vi "TurnOn.vi"(7 "Voltage Set (V)":dbl, 8 "error in (no error)":errorcluster, 9 "OCP Level (A)":dbl, 10 "OVP Level (V)":dbl, 11 "PSU_N87 in":refnum<class "PSU_N87.lvclass">) -> (0 "error out":errorcluster, 3 "PSU_N87 out":refnum<class "PSU_N87.lvclass">)   [LabVIEW 2014, in "PSU_N87.lvclass"]
uses:
  PSU_N87.lvclass
  PSU_N87.lvclass/PSU_N87.ctl
  PSU.lvclass
  <instrlib>/Agilent N87XX Series/Agilent N87XX Series.lvlib
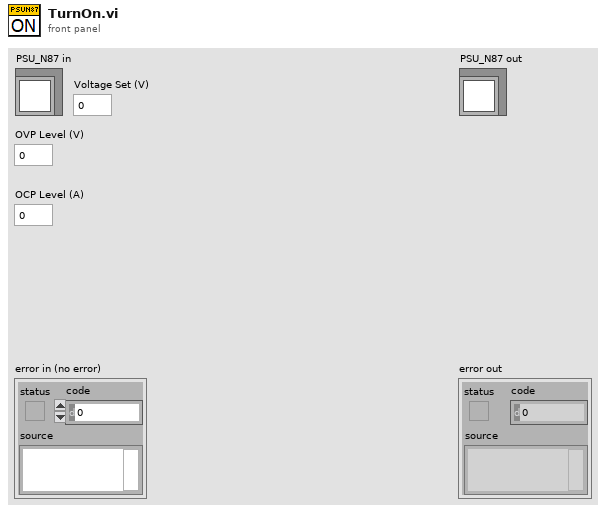
[diagram p1: front panel]
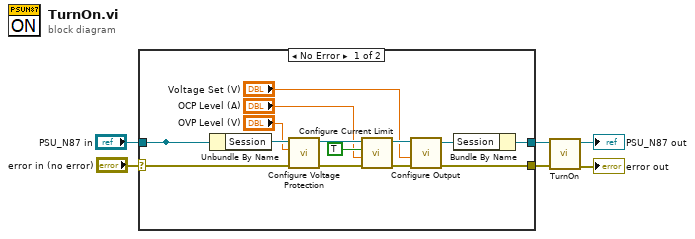
[diagram p0: block diagram]
diagram:
  n1 = case shown="No Error" "error in (no error)" {
    selector: "error in (no error)" -> [w15 w22]
    tunnel: [w14 w22] -> w3
    tunnel: "PSU_N87 in" -> [w12 w21]
    tunnel: [w7 w21] -> w4
    frame No Error {
      n2 = Unbundle By Name(w12) -> ("Session"=w13:refnum<visa-resource-name>)
      n3 = call <instrlib>:"Configure Voltage Protection.vi"("error in (no error)"=w15, "Over-Voltage Protection (5.0 V)"="OVP Level (V)", "VISA resource name"=w13) -> ("error out"=w16:errorcluster, "VISA resource name out"=w17:refnum<visa-resource-name>)  [unwired: 7 in]
      n4 = call <instrlib>:"Configure Current Limit.vi"("error in (no error)"=w16, "Current Limit (0.0 A)"="OCP Level (A)", "Enable Current Protection (F: Disable)"=TRUE, "VISA resource name"=w17) -> ("error out"=w18:errorcluster, "VISA resource name out"=w19:refnum<visa-resource-name>)  [unwired: 6 in]
      n5 = call <instrlib>:"Configure Output.vi"("error in (no error)"=w18, "Voltage Level (0.0 V)"="Voltage Set (V)", "VISA resource name"=w19) -> ("error out"=w14:errorcluster, "VISA resource name out"=w11:refnum<visa-resource-name>)  [unwired: 7 in]
      n6 = Bundle By Name(cluster=w12, "Session"=w11) -> (w7:refnum<class "PSU_N87.lvclass">)
    }
    frame Error {
    }
  }
  n7 = call-parent "TurnOn.vi"("error in (no error)"=w3, "PSU in"=w4) -> ("error out"=→"error out":errorcluster, "PSU out"=→"PSU_N87 out":refnum<class "PSU_N87.lvclass">)  [unwired: 8 in]
